vi "Get Data.vi"(8 "error in":errorcluster, 11 "Alicat Device in":refnum<class "Alicat Device.lvclass">) -> (0 "error out":errorcluster, 2 "Data":refnum<class "Data.lvclass">, 3 "Alicat Device out":refnum<class "Alicat Device.lvclass">)   [LabVIEW 2015, in "Alicat Lib.lvlib" / "Alicat Device.lvclass"]
doc: "Retrieve the data from the Alicat device. The Alicat device takes the address and returns data in a string format in the string <b>DataOut</b>. The data returned is also repackaged into the object <b>Alicat Data</b>."
uses:
  Alicat Device.lvclass
  <vilib>/MSR Consulting, LLC/General Reuse/Data/Data.lvclass
  <vilib>/MSR Consulting, LLC/Configurable Device/Configurable Device.lvclass/Configurable Device.ctl
  Alicat Device.lvclass/Alicat Device.ctl
  <vilib>/MSR Consulting, LLC/General Reuse/Data/Data.lvclass/Data.ctl
  Data/Alicat Data.lvclass/Alicat Data.ctl
  <vilib>/MSR Consulting, LLC/General Reuse/Data/Write Data ID.vi
  Data/Accessors/Write ID.vi
  <vilib>/MSR Consulting, LLC/Configurable Device/Read ID.vi
  Accessors/Read Alicat Data.vi
  <vilib>/MSR Consulting, LLC/General Reuse/Session APIs/Serial/Public/Get Data/Get String.vi
  Data/Alicat Data.lvclass
  <vilib>/MSR Consulting, LLC/General Reuse/Session APIs/Serial/Serial Session.lvclass
panel:
  out "DataOut":string
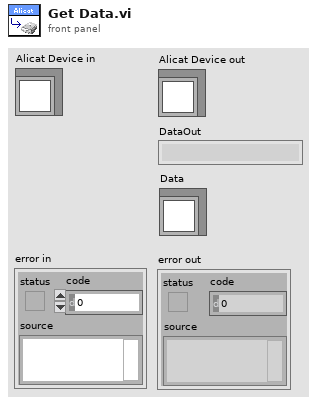
[diagram p1: front panel]
types:
  T1 = typedef "Serial Session.lvclass/Session Handle.ctl" = refnum<data-value>
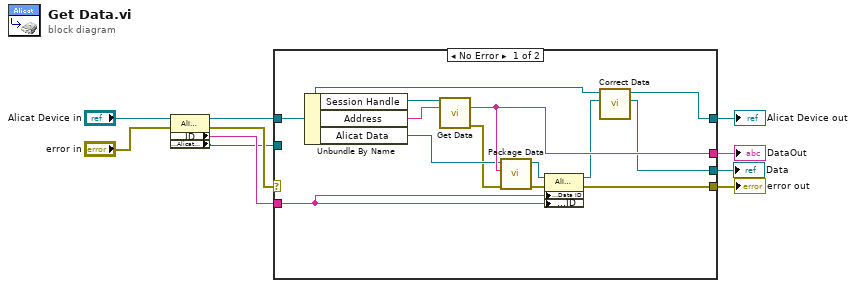
[diagram p0: block diagram]
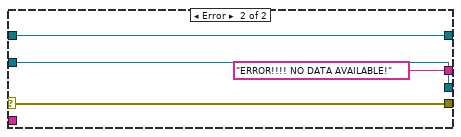
[diagram p2: hidden frame]
diagram:
  n1 = property class="Alicat Device"(reference="Alicat Device in", error in="error in") -> (reference out=w5:refnum<class "Alicat Device.lvclass">, error out=w3:errorcluster, "Accessors:ID"=w2:string, "Accessors:Alicat Data"=w1:refnum<class "Alicat Data.lvclass">)
  n2 = case shown="No Error" w3 {
    selector: w3 -> [_ w27]
    tunnel: w5 -> [w14 w26]
    tunnel: [w23 w27] -> w8
    tunnel: [w13 w26] -> w10
    tunnel: [w22 "ERROR!!!! NO DATA AVAILABLE!" ("DataOut")] -> w9
    tunnel: [w11 w24] -> w7
    tunnel: w2 -> [w21 _]
    tunnel: w1 -> [_ w24]
    frame No Error {
      n3 = Unbundle By Name(w14) -> ("Session Handle"=w20:T1, "Address"=w18:string, "Alicat Data"=w19:refnum<class "Alicat Data.lvclass">)
      n4 = call-poly <vilib>:"Get Data.vi"("Session Handle in"=w20, "CMD"=w18) -> ("DataOut"=w22:string, "error out"=w17:errorcluster)  [unwired: 11 in, 1 out]
      n5 = call-dynamic "Package Data.vi"("error in"=w17, "DataIn"=w22, "Alicat Data in"=w19) -> ("error out"=w15:errorcluster, "Alicat Data out"=w16:refnum<class "Alicat Data.lvclass">)  [unwired: 7 in]
      n6 = property class="Alicat Data"(reference=w16, error in=w15, "Accessors:Data ID"=w21, "Accessors:ID"=w21) -> (reference out=w12:refnum<class "Alicat Data.lvclass">, error out=w23:errorcluster)
      n7 = call-dynamic "Correct Data.vi"("Data In"=w12, "Alicat Device in"=w14) -> ("Data Out"=w11:refnum<class "Data.lvclass">, "Alicat Device out"=w13:refnum<class "Alicat Device.lvclass">)  [unwired: 7 in, 1 out]
    }
    frame Error {
    }
  }
  "error out" <- w8
  "Alicat Device out" <- w10
  "DataOut" <- w9
  "Data" <- w7
